vi "Emergency Broadcast.vi"(8 "error in (no error)":errorcluster, 9 "Mail Strategy In":refnum<class "Mail Strategy.lvclass">, 10 "Message In":refnum<class "Message.lvclass">, 11 "Simple Map Queue Group Messenger in":refnum<class "Simple Map Queue Group Messenger.lvclass">) -> (0 "error out":errorcluster, 3 "Simple Map Queue Group Messenger out":refnum<class "Simple Map Queue Group Messenger.lvclass">)   [LabVIEW 2024, in "Simple Map Queue Group Messenger.lvclass"]
uses:
  Simple Map Queue Group Messenger.lvclass
  Ancestor Class/Message/Message.lvclass
  Ancestor Class/Messenger/Mail Strategy/Mail Strategy.lvclass
  Simple Map Queue Group Messenger.lvclass/Simple Map Queue Group Messenger.ctl
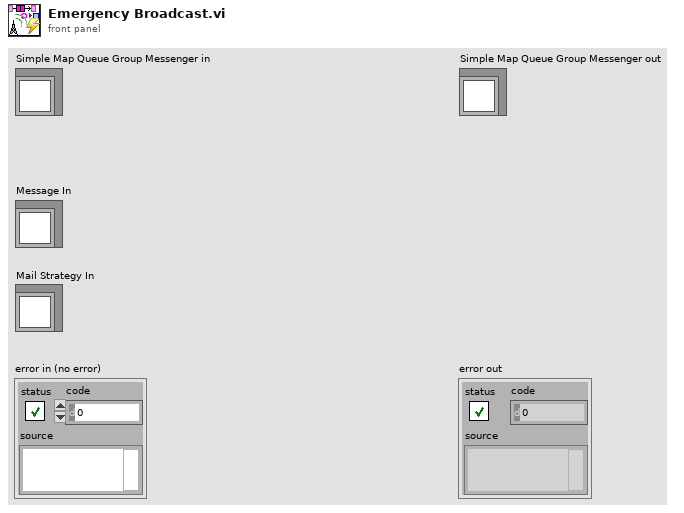
[diagram p1: front panel]
types:
  T1 = typedef "Queue Group Map.ctl" = map{i64, T2[]}
  T2 = typedef "Message Queue.ctl" = refnum<queue>
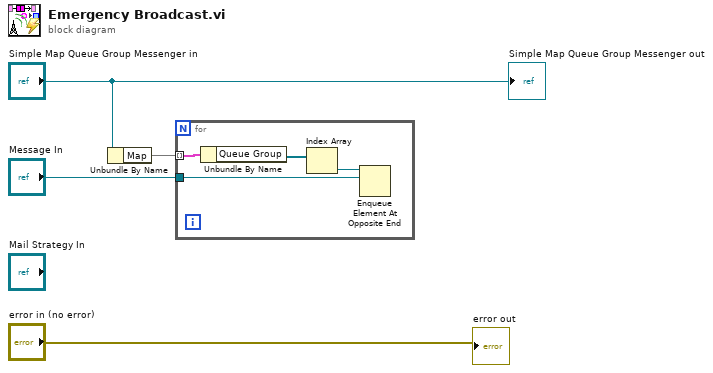
[diagram p0: block diagram]
diagram:
  n1 = Unbundle By Name("Simple Map Queue Group Messenger in") -> ("Map"=w4:T1)
  n2 = for {
    tunnel: w4 -> [w8] mode=indexing
    tunnel: "Message In" -> [w5]
    n3 = Unbundle By Name(w8) -> ("Queue Group"=w7:T2[])
    n4 = Index Array(array=w7) -> (element=w6:T2)  [unwired: 1 in]
    n5 = Enqueue Element At Opposite End(queue=w6, element=w5) -> ()  [unwired: 2 in, 3 out]
  }
  "error out" <- "error in (no error)"
  "Simple Map Queue Group Messenger out" <- "Simple Map Queue Group Messenger in"
